vi "GF_ConfigUSB6221.vi"(9 "QSwitch Delay":dbl=20.0, 10 "LaserClock \nFrequency":dbl=20.0) -> (0 "Laser Enable Channel":refnum<k21>, 1 "DO Clock":refnum<k21>="USB-MagAndTrigFire", 2 "LaserClock":refnum<k21>="USB-MagAndTrigFire", 3 "Fire Task":refnum<k21>="USB-MagAndTrigFire")   [LabVIEW 2016]
uses:
  <vilib>/DAQmx/write.llb/DAQmx Write (Counter Frequency 1Chan 1Samp).vi
  <vilib>/DAQmx/miscellaneous.llb/DAQmx Fill In Error Info.vi
  <vilib>/DAQmx/configure/timing.llb/DAQmx Timing (Sample Clock).vi
panel:
  out "LaserClock 2":refnum<k21>="USB-MagAndTrigFire"
  out "Measure Mag":refnum<k21>="USB-MagAndTrigFire"
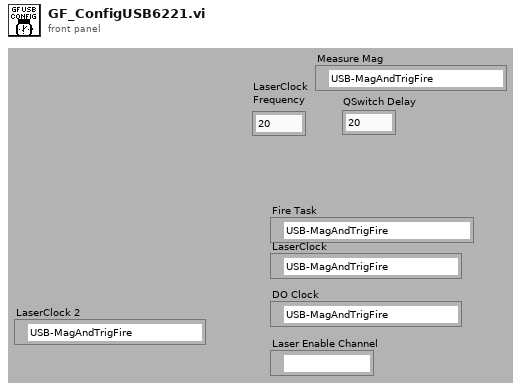
[diagram p1: front panel]
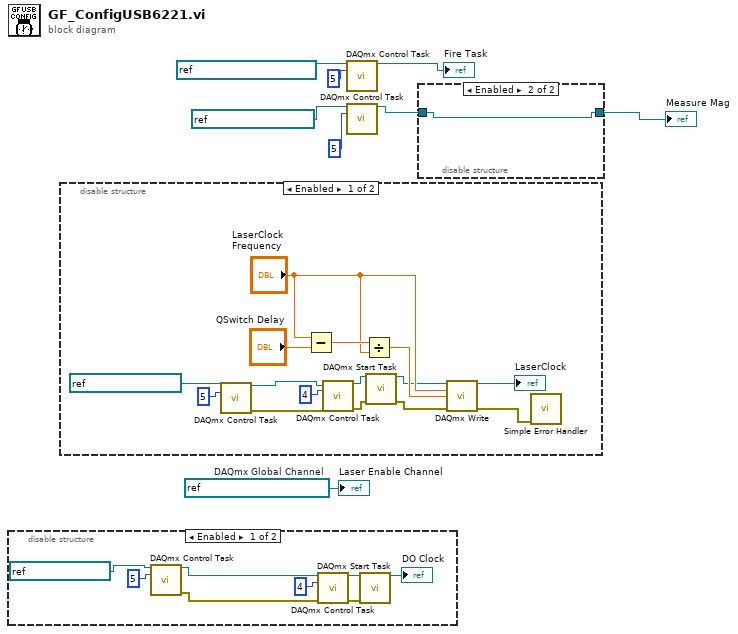
[diagram p0: block diagram]
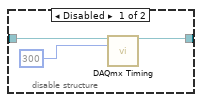
[diagram p2: hidden frame]
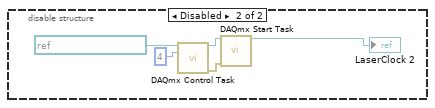
[diagram p3: hidden frame]
diagram:
  w8 = refnum<k21> "USB_LaserEnable_P0_6"  # DAQmx Global Channel
  n1 = disable-structure shown="Enabled" {
    frame Enabled {
      n2 = call <vilib>:"DAQmx Control Task.vi"("task/channels in"=refnum<k21> "USB-DOClock" ("DAQmx Task Name 3"), "action"=5) -> ("task out"=w12:refnum<k21>, "error out"=w10:errorcluster)  [unwired: 12 in]
      n3 = call <vilib>:"DAQmx Control Task.vi"("task/channels in"=w12, "action"=4, "error in"=w10) -> ("task out"=w15:refnum<k21>, "error out"=w9:errorcluster)  [unwired: 11 in]
      n4 = call <vilib>:"DAQmx Start Task.vi"("task/channels in"=w15, "error in"=w9) -> ("task out"=→"DO Clock":refnum<k21>)  [unwired: 12 in, 1 out]
    }
    frame Disabled {
    }
  }
  n5 = disable-structure shown="Enabled" {
    frame Enabled {
      n6 = call <vilib>:"DAQmx Control Task.vi"("task/channels in"=refnum<k21> "USB-LaserTimer" ("DAQmx Task Name 2"), "action"=5) -> ("task out"=w19:refnum<k21>, "error out"=w17:errorcluster)  [unwired: 12 in]
      n7 = Subtract(x="LaserClock \nFrequency", y="QSwitch Delay") -> (x-y=w28:dbl)
      n8 = call <vilib>:"DAQmx Control Task.vi"("task/channels in"=w19, "action"=4, "error in"=w17) -> ("task out"=w30:refnum<k21>, "error out"=w23:errorcluster)  [unwired: 11 in]
      n9 = Divide(x=w28, y="LaserClock \nFrequency") -> (x/y=w26:dbl)
      n10 = call <vilib>:"DAQmx Start Task.vi"("task/channels in"=w30, "error in"=w23) -> ("task out"=w25:refnum<k21>, "error out"=w22:errorcluster)  [unwired: 12 in]
      n11 = call-poly <vilib>:"DAQmx Write.vi"("task/channels in"=w25, "frequency"="LaserClock \nFrequency", "duty cycle"=w26, "error in"=w22) -> ("task out"=→"LaserClock":refnum<k21>, "error out"=w21:errorcluster)  [unwired: 9 in, 1 out]
      n12 = call <vilib>:"Simple Error Handler.vi"("error in (no error)"=w21) -> ()  [unwired: 4 in, 5 out]
    }
    frame Disabled {
      n13 = call <vilib>:"DAQmx Control Task.vi"("task/channels in"=refnum<k21> "USB-LaserTimer" ("DAQmx Task Name 2"), "action"=4) -> ("task out"=w34:refnum<k21>, "error out"=w32:errorcluster)  [unwired: 12 in]
      n14 = call <vilib>:"DAQmx Start Task.vi"("task/channels in"=w34, "error in"=w32) -> ("task out"=→"LaserClock 2":refnum<k21>)  [unwired: 12 in, 1 out]
    }
  }
  n15 = call <vilib>:"DAQmx Control Task.vi"("task/channels in"=refnum<k21> "USB-MagAndTrigFire" ("DAQmx Task Name"), "action"=5) -> ("task out"=→"Fire Task":refnum<k21>)  [unwired: 12 in, 1 out]
  n16 = call <vilib>:"DAQmx Control Task.vi"("task/channels in"=refnum<k21> "USB-MeasureMag" ("DAQmx Task Name 2"), "action"=5) -> ("task out"=w1:refnum<k21>)  [unwired: 12 in, 1 out]
  n17 = disable-structure shown="Enabled" {
    disable-tunnel: [w39 w40] -> w7
    disable-tunnel: w1 -> [w37 w40]
    frame Disabled {
      n18 = call-poly <vilib>:"DAQmx Timing.vi"("task/channels in"=w37, "rate"=300) -> ("task out"=w39:refnum<k21>)  [unwired: 12 in, 1 out]
    }
    frame Enabled {
    }
  }
  "Measure Mag" <- w7
  "Laser Enable Channel" <- w8
